vi "Refresh Database Import.vi"(8 "error in (no error)":errorcluster, 9 "Match settings":T1, 10 "DB":path=path "C:/Users/sbarrett/Desktop/Transfer Test.xml", 11 "Item Ref in":T2 format="%.0x") -> (0 "error out":errorcluster, 2 "DB dup":path=path "C:/Users/sbarrett/Desktop/Transfer Test.xml", 3 "Item Ref dup":T2 format="%.0x")   [LabVIEW 2012, in "AIT 429 System Explorer.lvlib"]
uses:
  AIT 429 System Explorer.lvlib
  <vilib>/NI Veristand/Custom Device API/Custom Device Item Ref.ctl
  Controls/Refresh Match Settings.ctl
  Create Sysdef Tree Labels.vi
  Build Label Properties.vi
  Refresh Param Channels.vi
  Refresh Default Value.vi
  Build Param Properties.vi
  Shared/Word to double.vi
  <vilib>/NI Veristand/Custom Device Tools/Custom Device Utility Library/NI VeriStand - Search for Item by GUID.vi
  Shared/Controls and Global/Global.vi
  <vilib>/NI Veristand/Custom Device Tools/Custom Device Utility Library/NI VeriStand - Search for Item by Name.vi
  <vilib>/NI Veristand/Custom Device Tools/Custom Device Utility Library/NI VeriStand - Search for Item by Property.vi
  <vilib>/NI Veristand/Custom Device API/NI VeriStand - Add Custom Device Section.vi
  AddParamChannels.vi
  <vilib>/NI Veristand/Custom Device API/NI VeriStand - Add Custom Device Channel.vi
  <vilib>/NI Veristand/Custom Device API/Set Item Property (U16).vi
  <vilib>/NI Veristand/Custom Device Tools/Custom Device Utility Library/NI VeriStand - Search for All Items by Property.vi
  <vilib>/NI Veristand/Custom Device API/Get Item Property (U32).vi
  <vilib>/NI Veristand/Custom Device API/Get Item Property (Boolean).vi
  <vilib>/NI Veristand/Custom Device API/Set Item Property (Variant).vi
  <vilib>/NI Veristand/Custom Device Tools/Custom Device Utility Library/NI VeriStand - Search for All Items by GUID.vi
  <vilib>/NI Veristand/Custom Device API/NI VeriStand - Get Item GUID.vi
  <vilib>/NI Veristand/Custom Device API/NI VeriStand - Get Item Parent.vi
  <vilib>/NI Veristand/Custom Device API/NI VeriStand - Set Custom Device Channel Default Value.vi
  <vilib>/NI Veristand/Custom Device API/Get Item Property (Double).vi
  <vilib>/NI Veristand/Custom Device API/Get Item Property (I32).vi
  <vilib>/NI Veristand/Custom Device API/Get Item Property (U16).vi
  <vilib>/NI Veristand/Custom Device Tools/Custom Device Utility Library/Custom Device Utility Library.lvlib
  ARINC 429 Shared.lvlib
  <vilib>/NI Veristand/Custom Device API/Custom Device API.lvlib
panel:
  out "Refreshing Database":i32(slide) scale=0.0..100.0
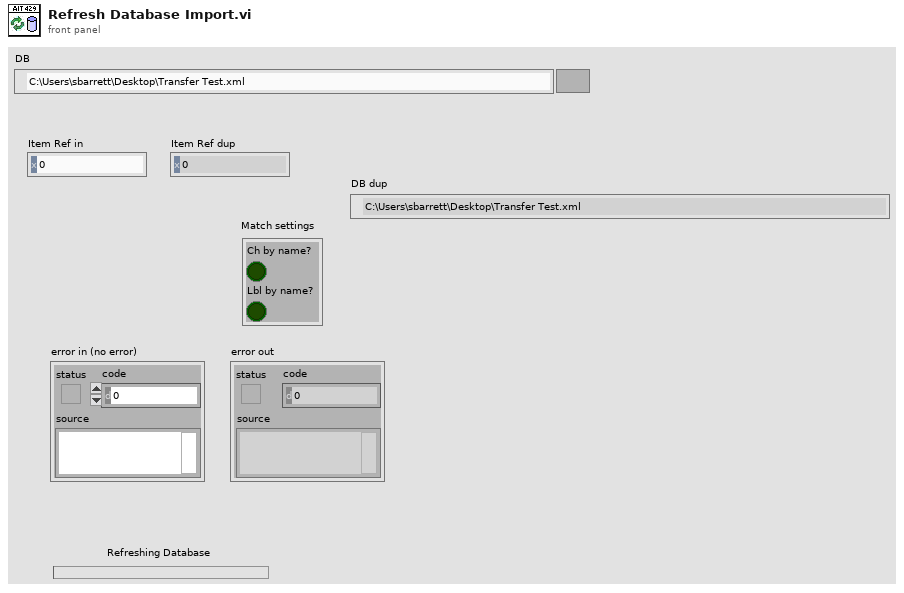
[diagram p1: front panel]
types:
  T1 = typedef "AIT 429 System Explorer.lvlib/Refresh Match Settings.ctl" = cluster{"Ch by name?":bool, "Lbl by name?":bool}
  T2 = typedef "Custom Device API.lvlib/Custom Device Item Ref.ctl" = u64
  T3 = enum16{"OWL429_DIRECTION_RX", "OWL429_DIRECTION_TX"}[]
  T4 = enum16{"OWL429_DIRECTION_RX", "OWL429_DIRECTION_TX"}
  T5 = typedef "AIT 429 System Explorer.lvlib/AIT_Channel Array.ctl" = T6[]
  T6 = typedef "AIT 429 System Explorer.lvlib/AIT_Channel.ctl" = cluster{"Labels":T7[], "name":string, "number":u8, "direction":enum16{"OWL429_DIRECTION_RX", "OWL429_DIRECTION_TX"}, "Voltage":dbl, "speed":T11}
  T7 = typedef "AIT 429 System Explorer.lvlib/AIT_Label.ctl" = cluster{"name":string, "xmlName":string, "TxPeriod":u32, "label":u32, "TxRate":dbl, "SDI_Enabled":bool, "SDIValue":u8, "BufferSize":u32, "Words":T8[], "TransferType":T10}
  T8 = typedef "AIT 429 System Explorer.lvlib/AIT_Word.ctl" = cluster{"InitalValue":u32, "Params":T9[]}
  T9 = typedef "AIT 429 System Explorer.lvlib/ARINCParam.ctl" = cluster{"name":string, "startBit":i32, "numberBits":i32, "scaleFactor":dbl, "scaleOffset":dbl, "signed":bool}
  T10 = typedef "ARINC 429 Shared.lvlib/TransferType.ctl" = enum16{"ScheduledLabel", "Acyclic", "Block", "Strobe"}
  T11 = typedef "Owl429.lvlib/Owl429ChannelSpeed.ctl" = enum16{"OWL429_HIGH_SPEED_CHANNEL", "OWL429_LOW_SPEED_CHANNEL"}
  T12 = typedef "Custom Device API.lvlib/Custom Device Item Info.ctl" = cluster{"Name":string, "Is Channel":bool, "GUID":string, "Is Waveform":bool}
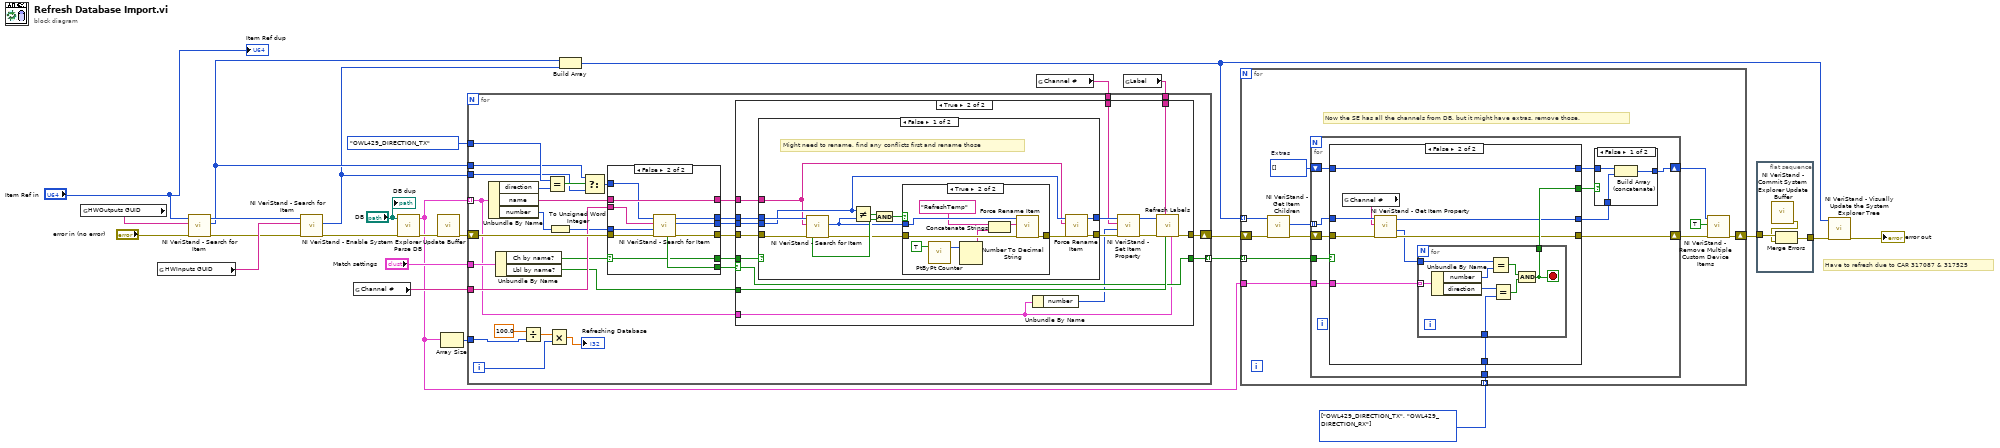
[diagram p0: block diagram]
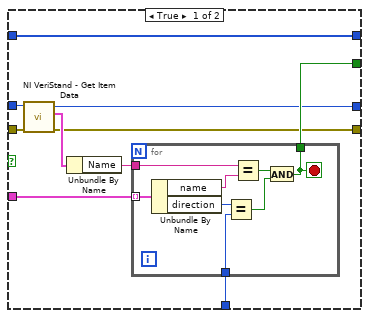
[diagram p3: hidden frame]
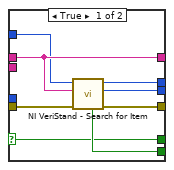
[diagram p4: hidden frame]
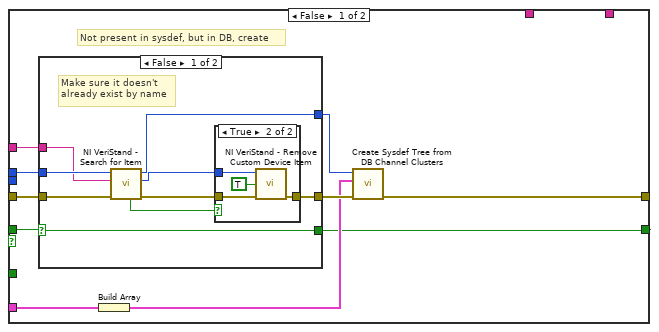
[diagram p5: hidden frame]
diagram:
  w11 = T3 [enum."OWL429_DIRECTION_TX", enum."OWL429_DIRECTION_RX"] items=["OWL429_DIRECTION_RX", "OWL429_DIRECTION_TX"]
  # "Have to refresh due to CAR 317087 & 317525"
  n1 = global read "Global.vi" "HWOutputs GUID"() -> (w26:string)
  n2 = global read "Global.vi" "HWInputs GUID"() -> (w24:string)
  n3 = call-poly <vilib>:"NI VeriStand - Search for Item.vi"("error in"="error in (no error)", "Item GUID"=w26, "Section Ref in"="Item Ref in") -> ("error out"=w23:errorcluster, "Item Ref"=w14:T2, "Section Ref out"=w25:T2)  [unwired: 5 in, 1 out]
  n4 = call-poly <vilib>:"NI VeriStand - Search for Item.vi"("error in"=w23, "Item GUID"=w24, "Section Ref in"=w25) -> ("error out"=w22:errorcluster, "Item Ref"=w13:T2)  [unwired: 5 in, 2 out]
  n5 = global read "Global.vi" "Channel #"() -> (w19:string)
  n6 = call "Parse DB.vi"("error in (no error)"=w22, "Path in"="DB") -> ("error out"=w17:errorcluster, "channels"=w2:T5)  [unwired: 8 in]
  n7 = call <vilib>:"NI VeriStand - Enable System Explorer Update Buffer.vi"("error in (no error)"=w17) -> ("error out"=w18:errorcluster)  [unwired: 10 in]
  n8 = Array Size(array=w2) -> (size(s)=w1:i32)
  n9 = Build Array(w14, w13) -> (w7:T2[])
  n10 = global read "Global.vi" "Channel #"() -> (w10:string)
  n11 = global read "Global.vi" "Label"() -> (w16:string)
  n12 = for {
    shift-right: [w39] -> w15
    shift-left: w18 -> [w56]
    tunnel: w2 -> [w34] mode=indexing
    tunnel: w13 -> [w51]
    tunnel: w14 -> [w50]
    tunnel: T4."OWL429_DIRECTION_TX" ("x") -> [w52]
    tunnel: "Match settings" -> [w45]
    tunnel: w19 -> [w44]
    tunnel: w16 -> [w35]
    tunnel: [w33] -> w12 mode=indexing
    tunnel: w10 -> [w32]
    tunnel: w1 -> [w30]
    i -> [w28]
    n13 = Unbundle By Name(w34) -> ("direction"=w55:T4, "name"=w53:string, "number"=w43:u8)
    n14 = Unbundle By Name(w45) -> ("Ch by name?"=w37:bool, "Lbl by name?"=w36:bool)
    n15 = Divide(x=100.0, y=w30) -> (x/y=w29:dbl)
    n16 = Equal?(x=w52, y=w55) -> (x = y?=w54:bool)
    n17 = Multiply(x=w29, y=w28) -> (x*y=→"Refreshing Database":dbl)
    n18 = To Unsigned Word Integer(number=w43) -> (unsigned 16bit integer=w38:u16)
    n19 = Select(t=w50, s=w54, f=w51) -> (s? t:f=w49:T2)
    n20 = case shown="False" w37 {
      selector: w37 -> [w58 w66]
      tunnel: w56 -> [w64 w74]
      tunnel: w53 -> [w59 w67]
      tunnel: w49 -> [w57 w65]
      tunnel: [w63 w73] -> w48
      tunnel: [w62 w72] -> w47
      tunnel: [w61 w71] -> w46
      tunnel: w44 -> [_ w70]
      tunnel: w38 -> [_ w69]
      tunnel: [w60 w68] -> w42
      tunnel: [w59 w67] -> w41
      tunnel: [w58 w66] -> w40
      frame True {
        n21 = call-poly <vilib>:"NI VeriStand - Search for Item.vi"("error in"=w64, "Item Name"=w59, "Section Ref in"=w57) -> ("error out"=w62:errorcluster, "Item Ref"=w61:T2, "Section Ref out"=w60:T2, "Found"=w63:bool)  [unwired: 5 in]
      }
      frame False {
        n22 = call-poly <vilib>:"NI VeriStand - Search for Item.vi"("error in"=w74, "Property Value"=w69, "Property Name"=w70, "Section Ref in"=w65) -> ("error out"=w72:errorcluster, "Item Ref"=w71:T2, "Section Ref out"=w68:T2, "Found"=w73:bool)  [unwired: 4 in]
      }
    }
    n23 = case shown="True" w48 {
      selector: w48 -> [_ w109]
      tunnel: w47 -> [w84 w112]
      tunnel: w46 -> [_ w113]
      tunnel: w42 -> [w83 w114]
      tunnel: w41 -> [w82 w110]
      tunnel: w40 -> [w81 w111]
      tunnel: w34 -> [w79 w103]
      tunnel: [w77 w116] -> w39
      tunnel: w36 -> [_ w115]
      tunnel: w35 -> [_ w117]
      tunnel: [w75 w109] -> w33
      tunnel: w32 -> [_ w104]
      frame False {
        # "Not present in sysdef, but in DB, create"
        n24 = case shown="False" w81 {
          selector: w81 -> [w86 w99]
          tunnel: w84 -> [w93 w101]
          tunnel: w83 -> [w92 w100]
          tunnel: w82 -> [w91 _]
          tunnel: [w88 w101] -> w80
          tunnel: [w87 w100] -> w76
          tunnel: [w86 w99] -> w75
          frame False {
            # "Make sure it doesn't\nalready exist by name"
            n25 = call-poly <vilib>:"NI VeriStand - Search for Item.vi"("error in"=w93, "Item Name"=w91, "Section Ref in"=w92) -> ("error out"=w90:errorcluster, "Item Ref"=w89:T2, "Section Ref out"=w87:T2, "Found"=w85:bool)  [unwired: 5 in]
            n26 = case shown="True" w85 {
              tunnel: w90 -> [w94 w98]
              tunnel: w89 -> [_ w97]
              tunnel: [w94 w95] -> w88
              frame False {
              }
              frame True {
                n27 = call <vilib>:"NI VeriStand - Remove Custom Device Item.vi"("error in (no error)"=w98, "Force Delete (F)"=TRUE, "Item Ref in"=w97) -> ("error out"=w95:errorcluster)  [unwired: 7 in, 1 out]
              }
            }
          }
          frame True {
          }
        }
        n28 = Build Array(w79) -> (w78:T6[])
        n29 = call "Create Sysdef Tree from DB Channel Clusters.vi"("error in"=w80, "Channels to create"=w78, "Device Ptr"=w76) -> ("error out"=w77:errorcluster)  [unwired: 7 in, 1 out]
      }
      frame True {
        n30 = case shown="False" w111 {
          tunnel: w112 -> [w128 w140]
          tunnel: w113 -> [w120 w139]
          tunnel: [w129 w140] -> w106
          tunnel: w114 -> [w127 _]
          tunnel: [w119 w139] -> w105
          tunnel: w110 -> [w118 _]
          frame False {
            # "Might need to rename, find any conflicts first and rename those"
            n31 = call-poly <vilib>:"NI VeriStand - Search for Item.vi"("error in"=w128, "Item Name"=w118, "Section Ref in"=w127) -> ("error out"=w123:errorcluster, "Item Ref"=w122:T2, "Found"=w125:bool)  [unwired: 5 in, 1 out]
            n32 = Not Equal?(x=w120, y=w122) -> (x != y?=w126:bool)
            n33 = And(x=w126, y=w125) -> (x .and. y?=w124:bool)
            n34 = case shown="True" w124 {
              tunnel: w123 -> [w130 w138]
              tunnel: w122 -> [_ w137]
              tunnel: [w130 w136] -> w121
              frame False {
              }
              frame True {
                n35 = call "PtByPt Counter.vi"("activate"=TRUE) -> ("counter"=w134:u32)  [unwired: 1 in, 1 out]
                n36 = Number To Decimal String(number=w134) -> (decimal integer string=w133:string)  [unwired: 1 in]
                n37 = Concatenate Strings("RefreshTemp", w133) -> (w131:string)
                n38 = call "Force Rename Item.vi"("error in"=w138, "String"=w131, "Item Ref"=w137) -> ("error out"=w136:errorcluster)  [unwired: 7 in, 1 out]
              }
            }
            n39 = call "Force Rename Item.vi"("error in"=w121, "String"=w118, "Item Ref"=w120) -> ("error out"=w129:errorcluster, "Item Ref out"=w119:T2)  [unwired: 7 in]
          }
          frame True {
            # "Item found by name, don't need to rename"
          }
        }
        n40 = Unbundle By Name(w103) -> ("number"=w102:u8)
        n41 = call-poly <vilib>:"NI VeriStand - Set Item Property.vi"("error in (no error)"=w106, "Value"=w102, "Property Name"=w104, "Item Ref in"=w105) -> ("error out"=w108:errorcluster, "Item Ref out"=w107:T2)  [unwired: 5 in, 1 out]
        n42 = call "Refresh Labels.vi"("channel"=w103, "Lbl by name?"=w115, "Label"=w117, "error in"=w108, "Item Ref"=w107) -> ("error out"=w116:errorcluster)  [unwired: 6 in]
      }
    }
  }
  n43 = for {
    shift-right: [w145] -> w6
    shift-left: w15 -> [w146]
    tunnel: w7 -> [w144] mode=indexing
    tunnel: w2 -> [w143]
    tunnel: w12 -> [w142] mode=indexing
    tunnel: w11 -> [w141] mode=indexing
    w149 = T2[] []  # Extras
    # "Now the SE has all the channels from DB, but it might have extras, remove those."
    n44 = call <vilib>:"NI VeriStand - Get Item Children.vi"("error in (no error)"=w146, "Item Ref in"=w144) -> ("error out"=w147:errorcluster, "Child Refs"=w148:T2[])  [unwired: 6 in, 2 out]
    n45 = for {
      shift-right: [w160] -> w150
      shift-left: w147 -> [w163]
      tunnel: w148 -> [w162] mode=indexing
      tunnel: w143 -> [w161]
      shift-right: [w156] -> w151
      shift-left: w149 -> [w159]
      tunnel: w142 -> [w154]
      tunnel: w141 -> [w153]
      n46 = case shown="False" w154 {
        tunnel: w163 -> [w177 w195]
        tunnel: w162 -> [w176 w194]
        tunnel: w161 -> [w174 w193]
        tunnel: [w172 w192] -> w158
        tunnel: [w171 w191] -> w160
        tunnel: w159 -> [w170 w190]
        tunnel: [w170 w190] -> w157
        tunnel: [w169 w189] -> w155
        tunnel: w153 -> [w168 w186]
        frame True {
          n47 = call <vilib>:"NI VeriStand - Get Item Data.vi"("error in (no error)"=w177, "Item Ref in"=w176) -> ("error out"=w171:errorcluster, "Item Info"=w175:T12, "Item Ref out"=w169:T2)  [unwired: 6 in, 1 out]
          n48 = Unbundle By Name(w175) -> ("Name"=w173:string)
          n49 = for {
            tunnel: w174 -> [w185] mode=indexing
            tunnel: w173 -> [w184]
            tunnel: [w178] -> w172
            tunnel: w168 -> [w181]
            stop <- w178 stop-if-true
            n50 = Unbundle By Name(w185) -> ("name"=w183:string, "direction"=w182:T4)
            n51 = Equal?(x=w182, y=w181) -> (x = y?=w180:bool)
            n52 = Equal?(x=w184, y=w183) -> (x = y?=w179:bool)
            n53 = And(x=w179, y=w180) -> (x .and. y?=w178:bool)
          }
        }
        frame False {
          n54 = global read "Global.vi" "Channel #"() -> (w188:string)
          n55 = call-poly <vilib>:"NI VeriStand - Get Item Property.vi"("error in (no error)"=w195, "Property Name"=w188, "Item Ref in"=w194) -> ("error out"=w191:errorcluster, "Value"=w187:u16, "Item Ref out"=w189:T2)  [unwired: 5 in, 1 out]
          n56 = for {
            tunnel: w193 -> [w203] mode=indexing
            tunnel: w187 -> [w201]
            tunnel: [w196] -> w192
            tunnel: w186 -> [w199]
            stop <- w196 stop-if-true
            n57 = Unbundle By Name(w203) -> ("number"=w202:u8, "direction"=w200:T4)
            n58 = Equal?(x=w201, y=w202) -> (x = y?=w198:bool)
            n59 = Equal?(x=w200, y=w199) -> (x = y?=w197:bool)
            n60 = And(x=w198, y=w197) -> (x .and. y?=w196:bool)
          }
        }
      }
      n61 = case shown="False" w158 {
        tunnel: w157 -> [w166 w167]
        tunnel: [w165 w167] -> w156
        tunnel: w155 -> [w164 _]
        frame False {
          n62 = Build Array (concatenate)(w166, w164) -> (w165:T2[])
        }
        frame True {
        }
      }
    }
    n63 = call <vilib>:"NI VeriStand - Remove Multiple Custom Device Items.vi"("error in (no error)"=w150, "Force Delete (F)"=TRUE, "Item Refs in"=w151) -> ("error out"=w145:errorcluster)  [unwired: 7 in, 1 out]
  }
  n64 = flat-sequence {
    tunnel: w6 -> [w206]
    tunnel: [w204] -> w4
    frame #0 {
      n65 = call <vilib>:"NI VeriStand - Commit System Explorer Update Buffer.vi"() -> ("error out"=w205:errorcluster)  [unwired: 11 in]
      n66 = Merge Errors(w206, w205) -> (w204:errorcluster)
    }
  }
  n67 = call "NI VeriStand - Visually Update the System Explorer Tree.vi"("error in (no error)"=w4, "Node IDs"=w7) -> ("error out"=→"error out":errorcluster)  [unwired: 9 in]
  "Item Ref dup" <- "Item Ref in"
  "DB dup" <- "DB"
